vi "Read_Holding_Register.vi"(10 "Escritura_Variables":u16[](array[numeric])) -> (1 "Registros_B":u16[](array[numeric]), 2 "Registros_A":u16[](array[numeric]), 3 "Variables_Lectura":u16[](array[numeric]))   [LabVIEW 2017, in "Lib_Maestro_Ingen.lvlib"]
uses:
  Lib_Maestro_Ingen.lvlib
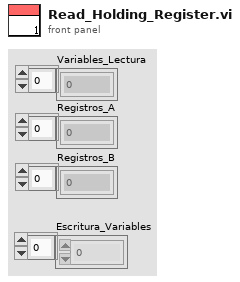
[diagram p1: front panel]
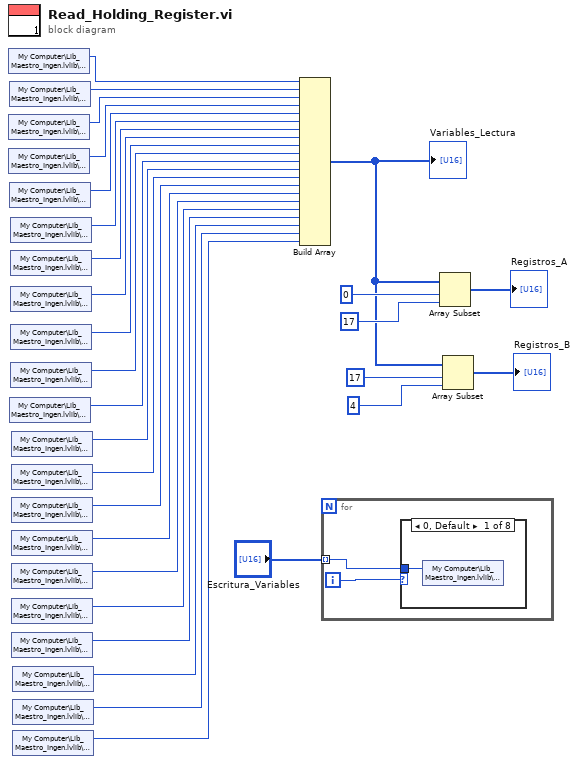
[diagram p0: block diagram]
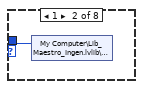
[diagram p2: hidden frame]
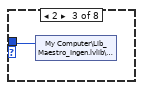
[diagram p3: hidden frame]
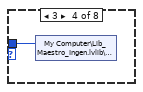
[diagram p4: hidden frame]
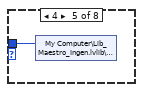
[diagram p5: hidden frame]
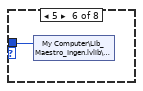
[diagram p6: hidden frame]
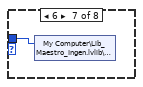
[diagram p7: hidden frame]
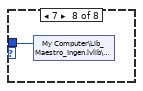
[diagram p8: hidden frame]
diagram:
  n1 = shared-variable "My Computer\\Lib_Maestro_Ingen.lvlib\\300001"() -> (w29:u16)  [unwired: 1 in, 1 out]
  n2 = shared-variable "My Computer\\Lib_Maestro_Ingen.lvlib\\300003"() -> (w27:u16)  [unwired: 1 in, 1 out]
  n3 = shared-variable "My Computer\\Lib_Maestro_Ingen.lvlib\\300004"() -> (w26:u16)  [unwired: 1 in, 1 out]
  n4 = shared-variable "My Computer\\Lib_Maestro_Ingen.lvlib\\300002"() -> (w28:u16)  [unwired: 1 in, 1 out]
  n5 = shared-variable "My Computer\\Lib_Maestro_Ingen.lvlib\\300005"() -> (w25:u16)  [unwired: 1 in, 1 out]
  n6 = shared-variable "My Computer\\Lib_Maestro_Ingen.lvlib\\300011"() -> (w19:u16)  [unwired: 1 in, 1 out]
  n7 = shared-variable "My Computer\\Lib_Maestro_Ingen.lvlib\\300006"() -> (w24:u16)  [unwired: 1 in, 1 out]
  n8 = shared-variable "My Computer\\Lib_Maestro_Ingen.lvlib\\300007"() -> (w23:u16)  [unwired: 1 in, 1 out]
  n9 = shared-variable "My Computer\\Lib_Maestro_Ingen.lvlib\\300008"() -> (w22:u16)  [unwired: 1 in, 1 out]
  n10 = shared-variable "My Computer\\Lib_Maestro_Ingen.lvlib\\300009"() -> (w21:u16)  [unwired: 1 in, 1 out]
  n11 = shared-variable "My Computer\\Lib_Maestro_Ingen.lvlib\\300010"() -> (w20:u16)  [unwired: 1 in, 1 out]
  n12 = shared-variable "My Computer\\Lib_Maestro_Ingen.lvlib\\300012"() -> (w18:u16)  [unwired: 1 in, 1 out]
  n13 = shared-variable "My Computer\\Lib_Maestro_Ingen.lvlib\\300013"() -> (w17:u16)  [unwired: 1 in, 1 out]
  n14 = shared-variable "My Computer\\Lib_Maestro_Ingen.lvlib\\300014"() -> (w16:u16)  [unwired: 1 in, 1 out]
  n15 = shared-variable "My Computer\\Lib_Maestro_Ingen.lvlib\\300015"() -> (w15:u16)  [unwired: 1 in, 1 out]
  n16 = shared-variable "My Computer\\Lib_Maestro_Ingen.lvlib\\300016"() -> (w14:u16)  [unwired: 1 in, 1 out]
  n17 = shared-variable "My Computer\\Lib_Maestro_Ingen.lvlib\\300017"() -> (w13:u16)  [unwired: 1 in, 1 out]
  n18 = shared-variable "My Computer\\Lib_Maestro_Ingen.lvlib\\300018"() -> (w12:u16)  [unwired: 1 in, 1 out]
  n19 = shared-variable "My Computer\\Lib_Maestro_Ingen.lvlib\\300019"() -> (w11:u16)  [unwired: 1 in, 1 out]
  n20 = shared-variable "My Computer\\Lib_Maestro_Ingen.lvlib\\300020"() -> (w10:u16)  [unwired: 1 in, 1 out]
  n21 = shared-variable "My Computer\\Lib_Maestro_Ingen.lvlib\\300021"() -> (w9:u16)  [unwired: 1 in, 1 out]
  n22 = Build Array(w29, w28, w27, w26, w25, w24, w23, w22, w21, w20, w19, w18, w17, w16, w15, w14, w13, w12, w11, w10, w9) -> (w6:u16[])
  "Variables_Lectura" <- w6
  n23 = for {
    tunnel: "Escritura_Variables" -> [w30] mode=indexing
    i -> [w31]
    n24 = case shown="0, Default" w31 {
      tunnel: w30 -> [w32 w33 w34 w35 w36 w37 w38 w39]
      frame 0, Default {
        n25 = shared-variable "My Computer\\Lib_Maestro_Ingen.lvlib\\300022"(w32) -> ()  [unwired: 1 in, 1 out]
      }
      frame 1 {
        n26 = shared-variable "My Computer\\Lib_Maestro_Ingen.lvlib\\300023"(w33) -> ()  [unwired: 1 in, 1 out]
      }
      frame 2 {
        n27 = shared-variable "My Computer\\Lib_Maestro_Ingen.lvlib\\300024"(w34) -> ()  [unwired: 1 in, 1 out]
      }
      frame 3 {
        n28 = shared-variable "My Computer\\Lib_Maestro_Ingen.lvlib\\300025"(w35) -> ()  [unwired: 1 in, 1 out]
      }
      frame 4 {
        n29 = shared-variable "My Computer\\Lib_Maestro_Ingen.lvlib\\300026"(w36) -> ()  [unwired: 1 in, 1 out]
      }
      frame 5 {
        n30 = shared-variable "My Computer\\Lib_Maestro_Ingen.lvlib\\300027"(w37) -> ()  [unwired: 1 in, 1 out]
      }
      frame 6 {
        n31 = shared-variable "My Computer\\Lib_Maestro_Ingen.lvlib\\300028"(w38) -> ()  [unwired: 1 in, 1 out]
      }
      frame 7 {
        n32 = shared-variable "My Computer\\Lib_Maestro_Ingen.lvlib\\300029"(w39) -> ()  [unwired: 1 in, 1 out]
      }
    }
  }
  n33 = Array Subset(array=w6, index=0, length=17) -> (→"Registros_A":u16[])
  n34 = Array Subset(array=w6, index=17, length=4) -> (→"Registros_B":u16[])
